vi "AUTON_Index.vi"(0 "Auton Array":dbl[][](array[numeric]), 5 "MeasuredHeading":dbl, 7 "LeftEncoder":dbl, 9 "RightEncoder":dbl, 11 "Kinect Array":dbl[](array[numeric])) -> (3 "Kinect Array Out":dbl[](array[numeric]), 4 "Left Drive":dbl, 6 "Right Drive":dbl)   [LabVIEW 2011]
uses:
  <vilib>/addons/Kinect/Skeleton Vertex Index.ctl
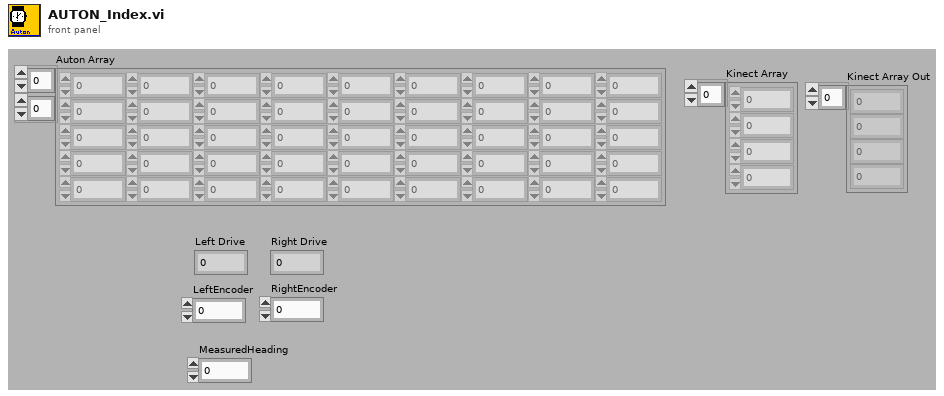
[diagram p1: front panel]
types:
  T1 = typedef "Skeleton Vertex Index.ctl" = i32
  T2 = cluster{"RightAxis":dbl, "LeftAxis":dbl, "RightHead":bool, "Left Head":bool, "Left Leg Out":bool, "Left Leg Forward":bool, "Left Leg Back":bool, "Right Leg Out":bool, "Right Leg Forward":bool, "Right Leg Back":bool}
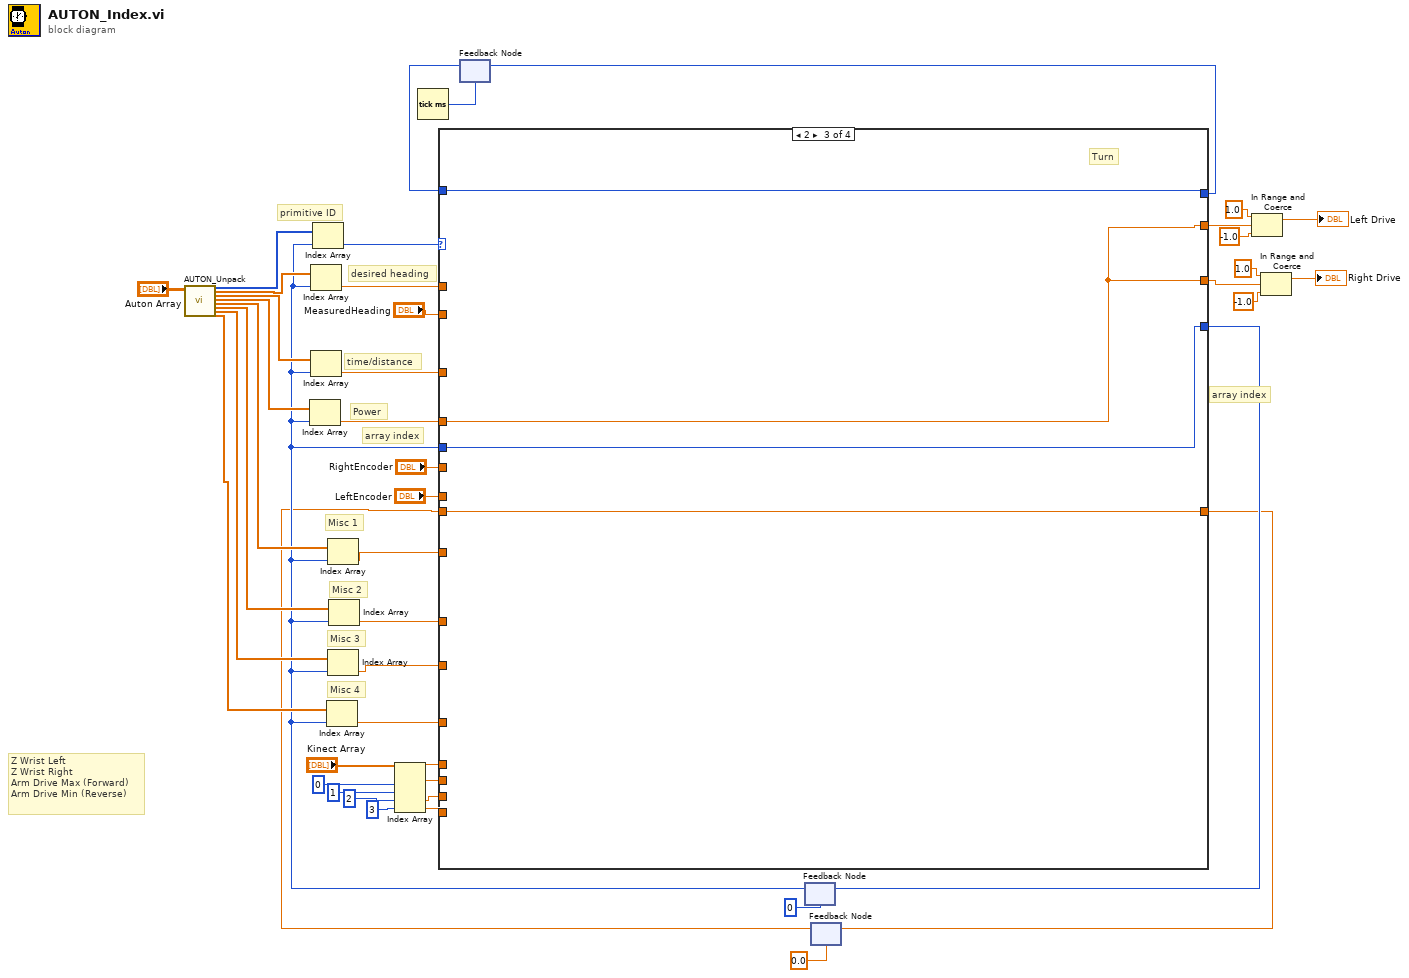
[diagram p0: block diagram]
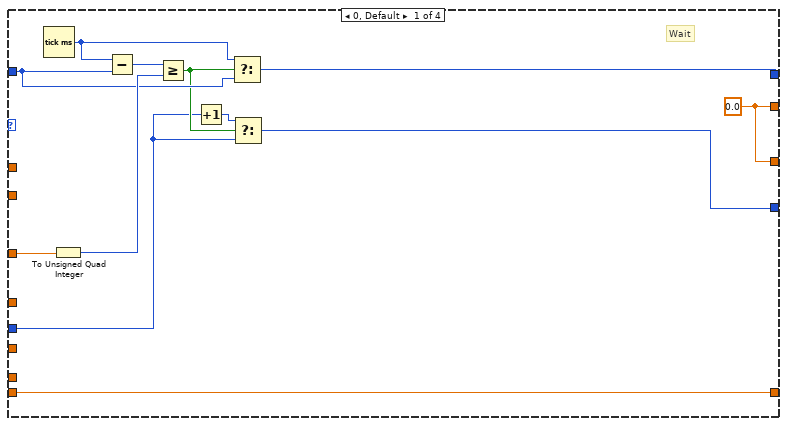
[diagram p2: hidden frame]
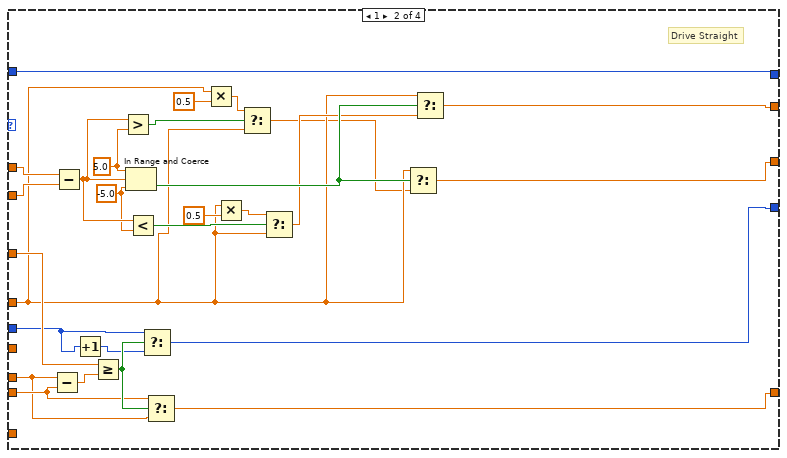
[diagram p3: hidden frame]
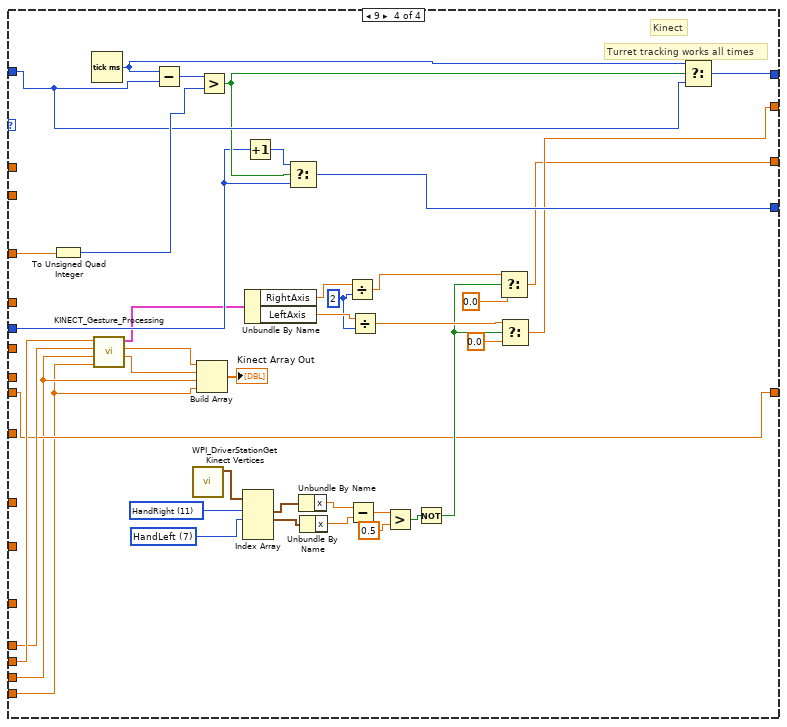
[diagram p4: hidden frame]
diagram:
  # "Misc 4"
  # "Misc 3"
  # "Misc 2"
  # "Misc 1"
  # "Z Wrist Left\nZ Wrist Right\nArm Drive Max (Forward)\nArm Drive Min (Reverse)"
  # "array index"
  # "array index"
  # "Power"
  # "desired heading"
  # "primitive ID"
  # "time/distance"
  n1 = call "AUTON_Unpack.vi"("all rows"="Auton Array") -> ("Primitive"=w45:i16[], "Desired Heading"=w24:dbl[], "Time/Distance"=w23:dbl[], "Power"=w22:dbl[], "Misc 1"=w21:dbl[], "Misc 2"=w20:dbl[], "Misc 3"=w19:dbl[], "Misc 4"=w18:dbl[])  [unwired: 1 in, 18 out]
  n2 = Index Array(array="Kinect Array", index #1=0 ("index"), index #2=1 ("index"), index #3=2 ("index"), index #4=3 ("index")) -> (element #1=w7:dbl, element #2=w6:dbl, element #3=w5:dbl, element #4=w4:dbl)
  n3 = Tick Count (ms)() -> (millisecond timer value=w40:u32)
  n4 = feedback #1(w40) -> (w44:u32)
  n5 = feedback #2(0) -> (w16:i32)
  n6 = Index Array(array=w22, index=w16) -> (element=w42:dbl)
  n7 = Index Array(array=w24, index=w16) -> (element=w29:dbl)
  n8 = Index Array(array=w23, index=w16) -> (element=w43:dbl)
  n9 = Index Array(array=w45, index=w16) -> (element=w26:i16)
  n10 = Index Array(array=w18, index=w16) -> (element=w17:dbl)
  n11 = Index Array(array=w21, index=w16) -> (element=w25:dbl)
  n12 = Index Array(array=w19, index=w16) -> (element=w14:dbl)
  n13 = Index Array(array=w20, index=w16) -> (element=w15:dbl)
  n14 = feedback #3(0.0) -> (w2:dbl)
  n15 = case shown="2" w26 {
    tunnel: [w50 w81 w87 w120] -> w27
    tunnel: w16 -> [w51 w61 w87 w121]
    tunnel: [w58 w63 w88 w128] -> w30
    tunnel: w44 -> [w55 w63 w88 w125]
    tunnel: w43 -> [w48 w83 _ w119]
    tunnel: w29 -> [_ w80 _ _]
    tunnel: [w49 w77 w89 w110] -> w38
    tunnel: [w49 w76 w89 w109] -> w31
    tunnel: w42 -> [_ w65 w89 _]
    tunnel: "LeftEncoder" -> [_ w59 _ _]
    tunnel: "MeasuredHeading" -> [_ w79 _ _]
    tunnel: w25 -> [_ _ _ _]
    tunnel: w17 -> [_ _ _ _]
    tunnel: w15 -> [_ _ _ _]
    tunnel: w14 -> [_ _ _ _]
    tunnel: "RightEncoder" -> [_ _ _ _]
    tunnel: w7 -> [_ _ _ w96]
    tunnel: w6 -> [_ _ _ w97]
    tunnel: w5 -> [_ _ _ w92]
    tunnel: w4 -> [_ _ _ w91]
    tunnel: w2 -> [w47 w60 w86 w95]
    tunnel: [w47 w85 w86 w95] -> w1
    frame 0, Default {
      w49 = 0.0 ("Numeric")
      # "Wait"
      n16 = Tick Count (ms)() -> (millisecond timer value=w54:u32)
      n17 = To Unsigned Quad Integer(1:w48) -> (0:w56:u64)
      n18 = Subtract(x=w54, y=w55) -> (x-y=w57:u32)
      n19 = Greater Or Equal?(x=w57, y=w56) -> (x >= y?=w53:bool)
      n20 = Increment(x=w51) -> (x+1=w52:i32)
      n21 = Select(t=w54, s=w53, f=w55) -> (s? t:f=w58:u32)
      n22 = Select(t=w52, s=w53, f=w51) -> (s? t:f=w50:i32)
    }
    frame 1 {
      w73 = -5.0 ("lower limit")
      w75 = 5.0 ("upper limit")
      # "Drive Straight"
      n23 = Subtract(x=w59, y=w60) -> (x-y=w84:dbl)
      n24 = Subtract(x=w80, y=w79) -> (x-y=w74:dbl)
      n25 = Increment(x=w61) -> (x+1=w62:i32)
      n26 = Greater Or Equal?(x=w83, y=w84) -> (x >= y?=w82:bool)
      n27 = Greater?(x=w74, y=w75) -> (0:w68:bool)
      n28 = In Range and Coerce(upper limit=w75, x=w74, lower limit=w73) -> (In Range?=w78:bool)  [unwired: 1 out]
      n29 = Less?(x=w74, y=w73) -> (x < y?=w72:bool)
      n30 = Select(t=w61, s=w82, f=w62) -> (s? t:f=w81:i32)
      n31 = Select(t=w60, s=w82, f=w59) -> (s? t:f=w85:dbl)
      n32 = Multiply(x=w65, y=0.5) -> (x*y=w67:dbl)
      n33 = Multiply(x=w65, y=0.5) -> (x*y=w70:dbl)
      n34 = Select(t=w67, s=w68, f=w65) -> (s? t:f=w64:dbl)
      n35 = Select(t=w70, s=w72, f=w65) -> (s? t:f=w69:dbl)
      n36 = Select(t=w65, s=w78, f=w64) -> (s? t:f=w76:dbl)
      n37 = Select(t=w65, s=w78, f=w69) -> (s? t:f=w77:dbl)
    }
    frame 2 {
      # "Turn"
    }
    frame 9 {
      w98 = T1 7 items=["HipCenter", "Spine", "ShoulderCenter", "Head", "ShoulderLeft", "ElbowLeft", "WristLeft", "HandLeft", "ShoulderRight", "ElbowRight", "WristRight", "HandRight", "HipLeft", "KneeLeft", "AnkleLeft", "FootLeft", "HipRight", "KneeRight", "AnkleRight", "FootRight"] ("Skeleton Joints")
      w100 = T1 11 items=["HipCenter", "Spine", "ShoulderCenter", "Head", "ShoulderLeft", "ElbowLeft", "WristLeft", "HandLeft", "ShoulderRight", "ElbowRight", "WristRight", "HandRight", "HipLeft", "KneeLeft", "AnkleLeft", "FootLeft", "HipRight", "KneeRight", "AnkleRight", "FootRight"] ("Skeleton Joints")
      w115 = 2
      # "Kinect"
      # "Turret tracking works all times"
      n38 = To Unsigned Quad Integer(1:w119) -> (0:w126:u64)
      n39 = Tick Count (ms)() -> (millisecond timer value=w124:u32)
      n40 = call "KINECT_Gesture_Processing.vi"("Z Wrist Right in"=w97, "Z Wrist Left in"=w96, "Arm Drive in Max (Forward)"=w92, "Arm Drive in Min (Reverse)"=w91) -> ("Joystick Data"=w118:T2, "Z Wrist Right out"=w94:dbl, "Z Wrist Left out"=w93:dbl)  [unwired: 2 in]
      n41 = Subtract(x=w124, y=w125) -> (x-y=w127:u32)
      n42 = call <vilib>:"WPI_DriverStationGet Kinect Vertices.vi"() -> ("Skeleton Vertices"=w108:cluster{"x":sgl, "y":sgl, "z":sgl}[])  [unwired: 10 in, 1 out]
      n43 = Build Array(w94, w93, w92, w91) -> (→"Kinect Array Out":dbl[])
      n44 = Greater?(x=w127, y=w126) -> (0:w123:bool)
      n45 = Index Array(array=w108, index #1=w100, index #2=w98) -> (element #1=w101:cluster{"x":sgl, "y":sgl, "z":sgl}, element #2=w99:cluster{"x":sgl, "y":sgl, "z":sgl})  [unwired: 2 in, 2 out]
      n46 = Increment(x=w121) -> (x+1=w122:i32)
      n47 = Unbundle By Name(w118) -> ("RightAxis"=w117:dbl, "LeftAxis"=w116:dbl)
      n48 = Select(t=w122, s=w123, f=w121) -> (s? t:f=w120:i32)
      n49 = Unbundle By Name(w101) -> ("x"=w107:sgl)
      n50 = Unbundle By Name(w99) -> ("x"=w106:sgl)
      n51 = Divide(x=w117, y=w115) -> (x/y=w114:dbl)
      n52 = Subtract(x=w107, y=w106) -> (x-y=w105:sgl)
      n53 = Divide(x=w116, y=w115) -> (x/y=w113:dbl)
      n54 = Greater?(x=w105, y=sgl 0.5) -> (0:w103:bool)
      n55 = Not(x=w103) -> (.not. x?=w102:bool)
      n56 = Select(t=w114, s=w102, f=0.0) -> (s? t:f=w109:dbl)
      n57 = Select(t=w113, s=w102, f=0.0) -> (s? t:f=w110:dbl)
      n58 = Select(t=w124, s=w123, f=w125) -> (s? t:f=w128:u32)
    }
  }
  n59 = feedback-in #1(w30) -> ()
  n60 = feedback-in #2(w27) -> ()
  n61 = feedback-in #3(w1) -> ()
  n62 = In Range and Coerce(upper limit=1.0, x=w38, lower limit=-1.0) -> (coerced(x)=→"Left Drive":dbl)  [unwired: 1 out]
  n63 = In Range and Coerce(upper limit=1.0, x=w31, lower limit=-1.0) -> (coerced(x)=→"Right Drive":dbl)  [unwired: 1 out]
